vi "Enumerate Canbus interfaces.vi"(11 "error in":errorcluster {"code" format="%.0x"}) -> (8 "Valid Canbus interfaces":string[](array[string]), 10 "Valid interface found":bool, 15 "error out":errorcluster)   [LabVIEW 2011]
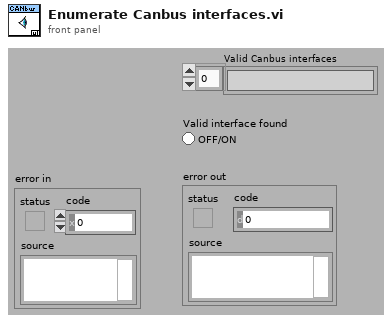
[diagram p1: front panel]
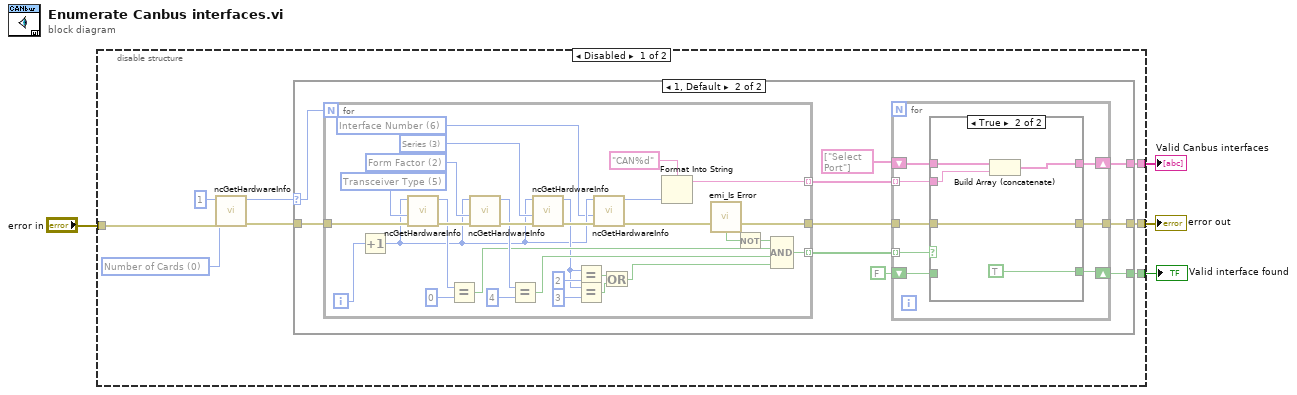
[diagram p0: block diagram]
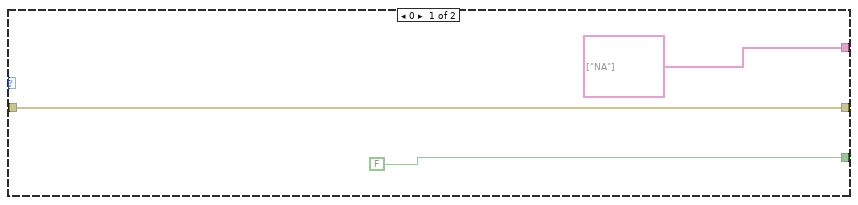
[diagram p2: hidden frame]
diagram:
  n1 = disable-structure shown="Disabled" {
    disable-tunnel: [w12 _] -> w4
    disable-tunnel: [w11 w72] -> w3
    disable-tunnel: "error in" -> [w10 w72]
    disable-tunnel: [w9 _] -> w1
    frame Disabled {
      w6 = u32 0 items=["Number of Cards", "Serial Number", "Form Factor", "Series", "Number of Ports", "Transceiver Type", "Interface Number", "Version Major", "Version Minor", "Version Update", "Version Phase", "Version Build", "Version Comment"] ("Attribute ID")
      n2 = call <vilib>:"ncGetHardwareInfo.vi"("error in"=w10, "Attribute ID"=w6, "card number"=u32 1) -> ("error out"=w8:errorcluster, "number"=w7:u32)  [unwired: 6 in, 1 out]
      n3 = case shown="1, Default" w7 {
        selector: w7 -> [_ w25]
        tunnel: w8 -> [w14 w24]
        tunnel: [FALSE w22] -> w9
        tunnel: [w14 w17] -> w11
        tunnel: [string[] ["NA"] w16] -> w12
        frame 0 {
        }
        frame 1, Default {
          n4 = for {
            N: w25 -> [_]
            tunnel: w24 -> [w70]
            tunnel: [w53] -> w21
            tunnel: [w50] -> w20 mode=indexing
            tunnel: [w44] -> w19 mode=indexing
            i -> [w71]
            w42 = u32 6 items=["Number of Cards", "Serial Number", "Form Factor", "Series", "Number of Ports", "Transceiver Type", "Interface Number", "Version Major", "Version Minor", "Version Update", "Version Phase", "Version Build", "Version Comment"] ("Attribute ID")
            w67 = u32 3 items=["Number of Cards", "Serial Number", "Form Factor", "Series", "Number of Ports", "Transceiver Type", "Interface Number", "Version Major", "Version Minor", "Version Update", "Version Phase", "Version Build", "Version Comment"] ("Attribute ID")
            w68 = u32 2 items=["Number of Cards", "Serial Number", "Form Factor", "Series", "Number of Ports", "Transceiver Type", "Interface Number", "Version Major", "Version Minor", "Version Update", "Version Phase", "Version Build", "Version Comment"] ("Attribute ID")
            w69 = u32 5 items=["Number of Cards", "Serial Number", "Form Factor", "Series", "Number of Ports", "Transceiver Type", "Interface Number", "Version Major", "Version Minor", "Version Update", "Version Phase", "Version Build", "Version Comment"] ("Attribute ID")
            n5 = Increment(x=w71) -> (x+1=w43:i32)
            n6 = call <vilib>:"ncGetHardwareInfo.vi"("error in"=w70, "Attribute ID"=w69, "card number"=w43) -> ("error out"=w66:errorcluster, "number"=w64:u32)  [unwired: 6 in, 1 out]
            n7 = Equal?(x=w64, y=u32 0) -> (x = y?=w54:bool)
            n8 = call <vilib>:"ncGetHardwareInfo.vi"("error in"=w66, "Attribute ID"=w68, "card number"=w43) -> ("error out"=w65:errorcluster, "number"=w62:u32)  [unwired: 6 in, 1 out]
            n9 = Equal?(x=w62, y=u32 4) -> (x = y?=w55:bool)
            n10 = call <vilib>:"ncGetHardwareInfo.vi"("error in"=w65, "Attribute ID"=w67, "card number"=w43) -> ("error out"=w49:errorcluster, "number"=w48:u32)  [unwired: 6 in, 1 out]
            n11 = Equal?(x=w48, y=u32 2) -> (x = y?=w57:bool)
            n12 = Equal?(x=w48, y=u32 3) -> (x = y?=w58:bool)
            n13 = call <vilib>:"ncGetHardwareInfo.vi"("error in"=w49, "Attribute ID"=w42, "card number"=w43) -> ("error out"=w45:errorcluster, "number"=w47:u32)  [unwired: 6 in, 1 out]
            n14 = Or(x=w57, y=w58) -> (x .or. y?=w56:bool)
            n15 = Format Into String(format string="CAN%d", w47) -> (resulting string=w44:string)  [unwired: 2 in, 1 out]
            n16 = call "emi_Is Error.vi"("error in (no error)"=w45) -> ("error out"=w53:errorcluster, "Is Error"=w52:bool)  [unwired: 13 in]
            n17 = Not(x=w52) -> (.not. x?=w51:bool)
            n18 = Compound Arithmetic op=AND(w51, w54, w55, w56) -> (w50:bool)
          }
          n19 = for {
            shift-right: [w31] -> w22
            shift-left: FALSE -> [w32]
            tunnel: w21 -> [w26]
            tunnel: w20 -> [w33] mode=indexing
            tunnel: w19 -> [w28] mode=indexing
            shift-right: [w29] -> w16
            shift-left: string[] ["Select Port"] -> [w30]
            tunnel: [w27] -> w17
            n20 = case shown="True" w33 {
              tunnel: w32 -> [w36 _]
              tunnel: [w36 TRUE] -> w31
              tunnel: w30 -> [w35 w40]
              tunnel: [w35 w39] -> w29
              tunnel: w28 -> [_ w38]
              tunnel: [w34 w37] -> w27
              tunnel: w26 -> [w34 w37]
              frame False {
              }
              frame True {
                n21 = Build Array (concatenate)(w40, w38) -> (w39:string[])
              }
            }
          }
        }
      }
    }
    frame Enabled {
    }
  }
  "Valid interface found" <- w1
  "error out" <- w3
  "Valid Canbus interfaces" <- w4
